vi "Cleanup.vi"(11 "Square":refnum<class "Square.lvclass">) -> ()   [LabVIEW 2020, in "SquareBattle.lvlib" / "Square.lvclass"]
doc: "This VI is called when a square is removed from the game. This can be due to collision, being attacked, or at the end of the game. If a square created any resources in Start, they should be cleaned up here. No further VIs will be called on the square once Cleanup is done."
uses:
  Square.lvclass
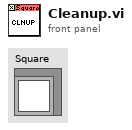
[diagram p1: front panel]
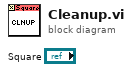
[diagram p0: block diagram]
diagram:
